vi "Update Meas Type to Repeat JV Scan for best.vi"(9 "Scan rate step number":dbl, 11 "Cell details array in":T1(array[cluster])) -> (3 "Cell details array out":T1(array[cluster]))   [LabVIEW 2016]
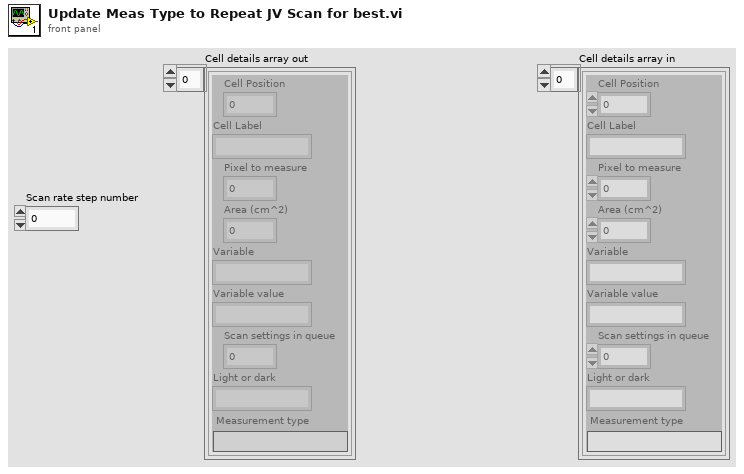
[diagram p1: front panel]
types:
  T1 = cluster{"Cell Position":i32, "Cell Label":string, "Pixel to measure":u16, "Area (cm^2)":dbl, "Variable":string, "Variable value":string, "Scan settings in queue":u16, "Light or dark":string, "Measurement type":string}[]
  T2 = cluster{"Cell Position":i32, "Cell Label":string, "Pixel to measure":u16, "Area (cm^2)":dbl, "Variable":string, "Variable value":string, "Scan settings in queue":u16, "Light or dark":string, "Measurement type":string}
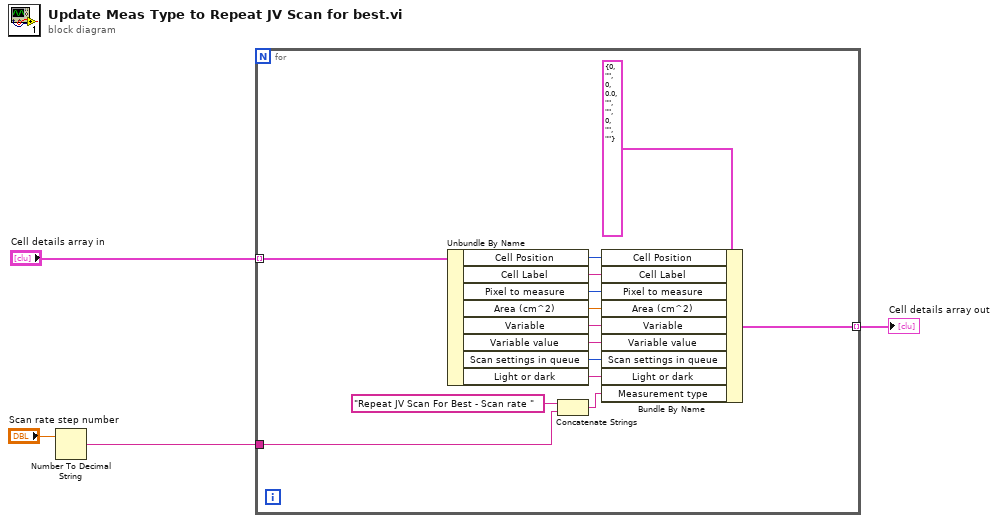
[diagram p0: block diagram]
diagram:
  n1 = Number To Decimal String(number="Scan rate step number") -> (decimal integer string=w1:string)  [unwired: 1 in]
  n2 = for {
    tunnel: "Cell details array in" -> [w18] mode=indexing
    tunnel: [w8] -> w3 mode=indexing
    tunnel: w1 -> [w6]
    n3 = Unbundle By Name(w18) -> ("Cell Position"=w16:i32, "Cell Label"=w15:string, "Pixel to measure"=w14:u16, "Area (cm^2)"=w13:dbl, "Variable"=w12:string, "Variable value"=w11:string, "Scan settings in queue"=w10:u16, "Light or dark"=w9:string)
    n4 = Concatenate Strings("Repeat JV Scan For Best - Scan rate " ("Measurement type"), w6) -> (w5:string)
    n5 = Bundle By Name(cluster=T2 {"Cell Position"=0, "Cell Label"="", "Pixel to measure"=0, "Area (cm^2)"=0.0, "Variable"="", "Variable value"="", "Scan settings in queue"=0, "Light or dark"="", "Measurement type"=""} ("Cluster"), "Cell Position"=w16, "Cell Label"=w15, "Pixel to measure"=w14, "Area (cm^2)"=w13, "Variable"=w12, "Variable value"=w11, "Scan settings in queue"=w10, "Light or dark"=w9, "Measurement type"=w5) -> (w8:T2)
  }
  "Cell details array out" <- w3
